vi "measure_aquisition_time.vi"(7 "Old Time / ms":u32) -> (8 "New Time / ms":u32, 12 "Aqusition Time / ms":u32, 14 "Aquisition Frequency / Hz":dbl)   [LabVIEW 2023]
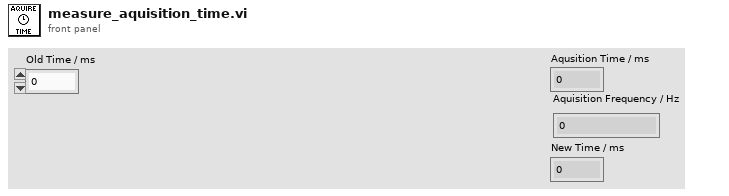
[diagram p1: front panel]
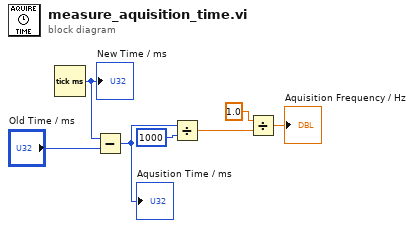
[diagram p0: block diagram]
diagram:
  n1 = Tick Count (ms)() -> (millisecond timer value=w6:u32)
  "New Time / ms" <- w6
  n2 = Subtract(x=w6, y="Old Time / ms") -> (x-y=w2:u32)
  "Aqusition Time / ms" <- w2
  n3 = Divide(x=w2, y=u32 1000) -> (x/y=w7:dbl)
  n4 = Divide(x=1.0, y=w7) -> (x/y=→"Aquisition Frequency / Hz":dbl)
